vi "Hand_Orientation.vi"(8 "Error In":errorcluster, 11 "Leap Handle in":T1) -> (0 "Error Out":errorcluster, 1 "Hand not tracked?":bool, 2 "Palm Orientation":dbl[](array[numeric]), 3 "Leap Handle":T1)   [LabVIEW 2015]
uses:
  <vilib>/MakerHub/Leap/Private/Type Defs/Leap Handle.ctl
  C:/Program Files (x86)/National Instruments/LabVIEW 2015/vi.lib/MakerHub/Leap/Private/Libs/LeapCSharp.NET3.5.dll
  Program Files (x86)/National Instruments/LabVIEW 2015/vi.lib/MakerHub/Leap/Private/Libs/LeapCSharp.NET3.5.dll
  <vilib>/MakerHub/Leap/LMH-Leap.lvlib
panel:
  # "Roll"
  # "Yaw"
  # "Pitch"
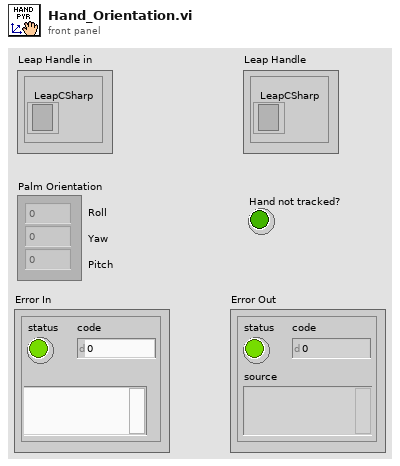
[diagram p1: front panel]
types:
  T1 = typedef "LMH-Leap.lvlib/Leap Handle.ctl" = cluster{"LeapCSharp":refnum<k24>}
  T2 = typedef "LMH-Leap.lvlib/Frame.ctl" = cluster{"ID":i64, "Timestamp":i64, "Current FPS":dbl, "Key Tap Gestures":T3[], "Circle Gestures":T8[], "Screen Tap Gestures":T9[], "Swipe Gestures":T10[], "Hands":T11[]}
  T3 = typedef "LMH-Leap.lvlib/Gesture Key Tap.ctl" = cluster{"Common":T4, "Direction":T7, "Position":T7, "Progress":dbl}
  T4 = typedef "LMH-Leap.lvlib/Gesture Common.ctl" = cluster{"ID":dbl, "Duration (S)":dbl, "Gesture Type":T5, "Gesture State":T6}
  T5 = typedef "LMH-Leap.lvlib/Gesture Type.ctl" = enum16{"Invalid", "Swipe", "Circle", "Screen Tap", "Key Tap"}
  T6 = typedef "LMH-Leap.lvlib/Gesture State.ctl" = enum16{"Invalid", "Start", "Update", "Stop"}
  T7 = typedef "LMH-Leap.lvlib/Vector.ctl" = cluster{"Pitch":sgl, "Yaw":sgl, "Roll":sgl, "Magnitude":sgl, "XYZ":sgl[]}
  T8 = typedef "LMH-Leap.lvlib/Gesture Circle.ctl" = cluster{"Common":T4, "Center":T7, "Normal":T7, "Progress":dbl, "Radius":dbl}
  T9 = typedef "LMH-Leap.lvlib/Gesture Screen Tap.ctl" = cluster{"Common":T4, "Direction":T7, "Position":T7, "Progress":dbl}
  T10 = typedef "LMH-Leap.lvlib/Gesture Swipe.ctl" = cluster{"Common":T4, "Direction":T7, "Position":T7, "Start Position":T7, "Speed":dbl}
  T11 = typedef "LMH-Leap.lvlib/Hand.ctl" = cluster{"Palm Normal":T7, "Palm Position":T7, "Palm Velocity":T7, "Direction":T7, "Palm Position (Stabilized)":T7, "Sphere Center":T7, "Pointables":T12[], "ID":i32, "Time Visible":sgl, "Sphere Radius":sgl}
  T12 = typedef "LMH-Leap.lvlib/Pointable.ctl" = cluster{"Type":T13, "Touch Zone":T14, "ID":i32, "Length":dbl, "Width":dbl, "Time Visible":dbl, "Touch Distance":dbl, "Direction":T7, "Tip Position":T7, "Tip Velocity":T7, "Tip Position (Stabilized)":T7}
  T13 = typedef "LMH-Leap.lvlib/Pointable Type.ctl" = enum16{"Finger", "Tool"}
  T14 = typedef "LMH-Leap.lvlib/Pointable Zone.ctl" = enum16{"None", "Hovering", "Touching"}
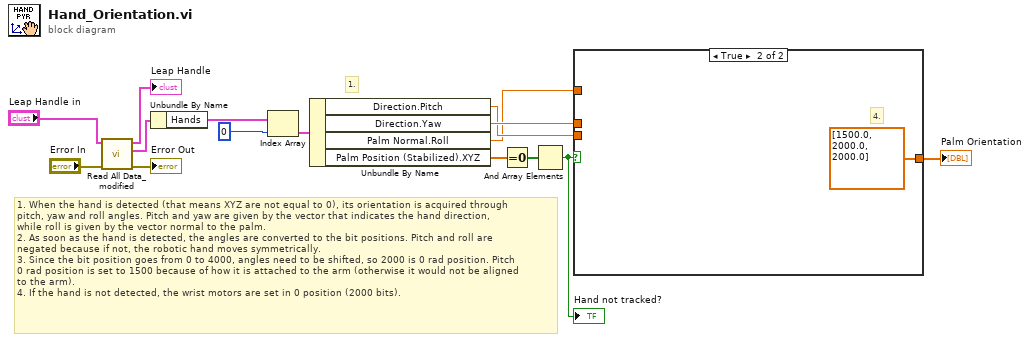
[diagram p0: block diagram]
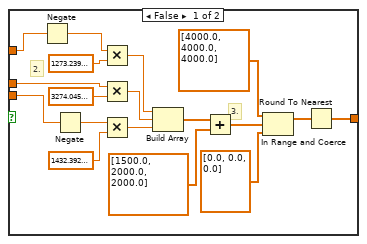
[diagram p2: hidden frame]
diagram:
  # "1."
  # "1. When the hand is detected (that means XYZ are not equal to 0), its orientation is acquired through \npitch, yaw and roll angles. Pitch and yaw are given by the vector that indicates the hand direction,\nwhile roll is given by the vector normal to the palm.\n2. As soon as the hand is detected, the angles are converted to the bit positions. Pitch and roll are \nnegated because if not, the robotic hand moves symmetrically.\n3. Since the bit position goes from 0 to 4000, angles need to be shifted, so 2000 is 0 rad position. Pitch\n0 rad position is set to 1500 because of how it is attached to the arm (otherwise it would not be aligned\nto the arm).\n4. If the hand is not detected, the wrist motors are set in 0 position (2000 bits)."
  n1 = call "Read All Data_modified.vi"("Error In"="Error In", "Leap Handle"="Leap Handle in") -> ("Error Out"=→"Error Out":errorcluster, "Frame"=w6:T2, "Leap Handle"=→"Leap Handle":T1)  [unwired: 6 in, 1 out]
  n2 = Unbundle By Name(w6) -> ("Hands"=w14:T11[])
  n3 = Index Array(array=w14, index=0) -> (element=w13:T11)
  n4 = Unbundle By Name(w13) -> ("Direction.Pitch"=w10:sgl, "Direction.Yaw"=w12:sgl, "Palm Normal.Roll"=w4:sgl, "Palm Position (Stabilized).XYZ"=w3:sgl[])
  n5 = Equal To 0?(x=w3) -> (x = 0?=w2:bool[])
  n6 = And Array Elements(Boolean array=w2) -> (logical AND=w1:bool)
  "Hand not tracked?" <- w1
  n7 = case shown="True" w1 {
    tunnel: w12 -> [w31 _]
    tunnel: [w20 sgl[] [1500.0, 2000.0, 2000.0]] -> w11
    tunnel: w10 -> [w19 _]
    tunnel: w4 -> [w17 _]
    frame False {
      # "3."
      # "2."
      n8 = Negate(x=w17) -> (-x=w16:sgl)
      n9 = Negate(x=w19) -> (-x=w18:sgl)
      n10 = Multiply(x=w16, y=sgl 1273.2395) -> (x*y=w27:sgl)
      n11 = Multiply(x=w31, y=sgl 3274.046) -> (x*y=w30:sgl)
      n12 = Multiply(x=w18, y=sgl 1432.3928) -> (x*y=w33:sgl)
      n13 = Build Array(w27, w30, w33) -> (w26:sgl[])
      n14 = Add(x=w26, y=sgl[] [1500.0, 2000.0, 2000.0]) -> (x+y=w24:sgl[])
      n15 = In Range and Coerce(upper limit=sgl[] [4000.0, 4000.0, 4000.0], x=w24, lower limit=sgl[] [0.0, 0.0, 0.0]) -> (coerced(x)=w21:sgl[])  [unwired: 1 out]
      n16 = Round To Nearest(number=w21) -> (nearest integer value=w20:sgl[])
    }
    frame True {
      # "4."
    }
  }
  "Palm Orientation" <- w11
